vi "Send Dialog Return Msg.vi"(8 "error in (no error)":errorcluster, 11 "Dialog Return Msg":refnum<class "Dialog Return Msg.lvclass">) -> (0 "error out":errorcluster)   [LabVIEW 2020, in "MVA Framework.lvlib" / "IDialogBox.lvlib" / "Dialog Return Msg.lvclass"]
doc: "<License>\nCopyright © 2017 Composed Systems, LLC | All rights reserved\nwww.composed.io\n\nAuthor: Ethan Stern <ethan.stern@composed.io>\n\nThis software is provided \"AS IS\" WITHOUT WARRANTIES, either express or implied, AND IS FOR EDUCATIONAL PURPOSES ONLY.\n</License>"
uses:
  Dialog Return Msg.lvclass
  Dialog Return Msg.lvclass/Dialog Return Msg.ctl
  <vilib>/ActorFramework/Message Enqueuer/Message Enqueuer.lvclass/Message Enqueuer.ctl
  <vilib>/ActorFramework/Message Priority Queue/Priority Enqueue.vi
  <vilib>/ActorFramework/Message Enqueuer/Message Enqueuer.lvclass
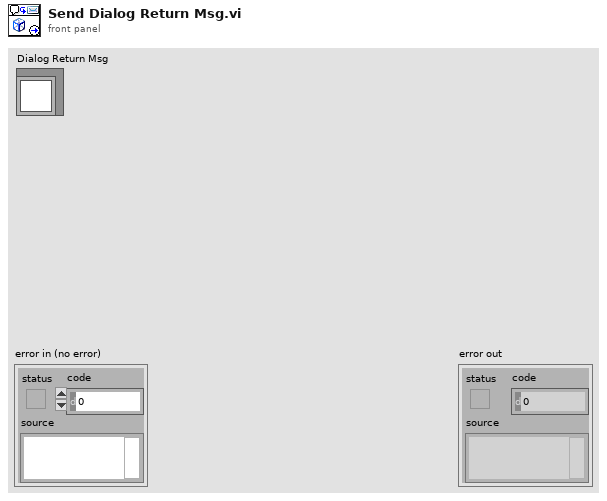
[diagram p1: front panel]
types:
  T1 = typedef "Actor Framework.lvlib/Message Enqueuer.lvclass/Message Priority.ctl" = enum16{"Low", "Normal", "High"}
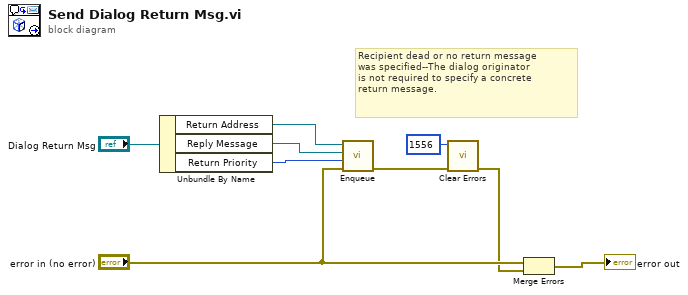
[diagram p0: block diagram]
diagram:
  # "Recipient dead or no return message\nwas specified--The dialog originator\nis not required to specify a concrete\nreturn message."
  n1 = Unbundle By Name("Dialog Return Msg") -> ("Return Address"=w7:refnum<class "Message Enqueuer.lvclass">, "Reply Message"=w8:refnum<class "Message.lvclass">, "Return Priority"=w6:T1)
  n2 = call <vilib>:"Enqueue.vi"("error in (no error)"="error in (no error)", "Message Priority (Normal)"=w6, "Message"=w8, "Message Enqueuer in"=w7) -> ("error out"=w4:errorcluster)  [unwired: 6 in, 1 out]
  n3 = call <vilib>:"Clear Errors.vi"("error in (no error)"=w4, "specific error code to clear (0: all)"=1556) -> ("error out"=w1:errorcluster)  [unwired: 4 in, 1 out]
  n4 = Merge Errors("error in (no error)", w1) -> (→"error out":errorcluster)
